vi "Init Deploy.vi"(8 "error in":errorcluster, 10 "Deployment Configuration":T6, 11 "simulator":T2) -> (2 "Communication Refs":T1[](array[typedef]), 3 "Remote Session List":refnum<k21>[](array[refnum]))   [LabVIEW 2014]
uses:
  Deployment  Configuration.ctl
  simulation/Simulator.ctl
  CyberSim interface/Simulation Configuration.ctl
  autograder/feedbackMode.ctl
  RobotData.ctl
  <instrlib>/DC Motor Controller/HAIOL/DC Motor Controller.lvclass
  iRobot Remote Ref.ctl
  iRobot/Sensor/Sensor Group 6.ctl
  iRobot/Sensor/Bumps + Wheel Drops.ctl
  iRobot/Sensor/Buttons.ctl
  iRobot/Sensor/Charging State.ctl
  iRobot/Sensor/Charging Sources Available.ctl
  iRobot/Sensor/OI Mode.ctl
  iRobot/Sensor/Cargo Bay Digital Inputs.ctl
  iRobot/Sensor/Low-Side Driver + Wheel Overcurrent.ctl
  <resource>/objmgr/nisysapi.rc
panel:
  # "Electrical: charging, battery, OI mode"
  # "Sensors: bump, cliff, button, wheel drop, wall, virtual wall"
  # "Motion: distance, angle, requested velocity"
  # "Cargo Bay: I/O, overcurrent, infrared"
  # "Song"
  # "Electrical: charging, battery, OI mode"
  # "Sensors: bump, cliff, button, wheel drop, wall, virtual wall"
  # "Motion: distance, angle, requested velocity"
  # "Cargo Bay: I/O, overcurrent, infrared"
  # "Song"
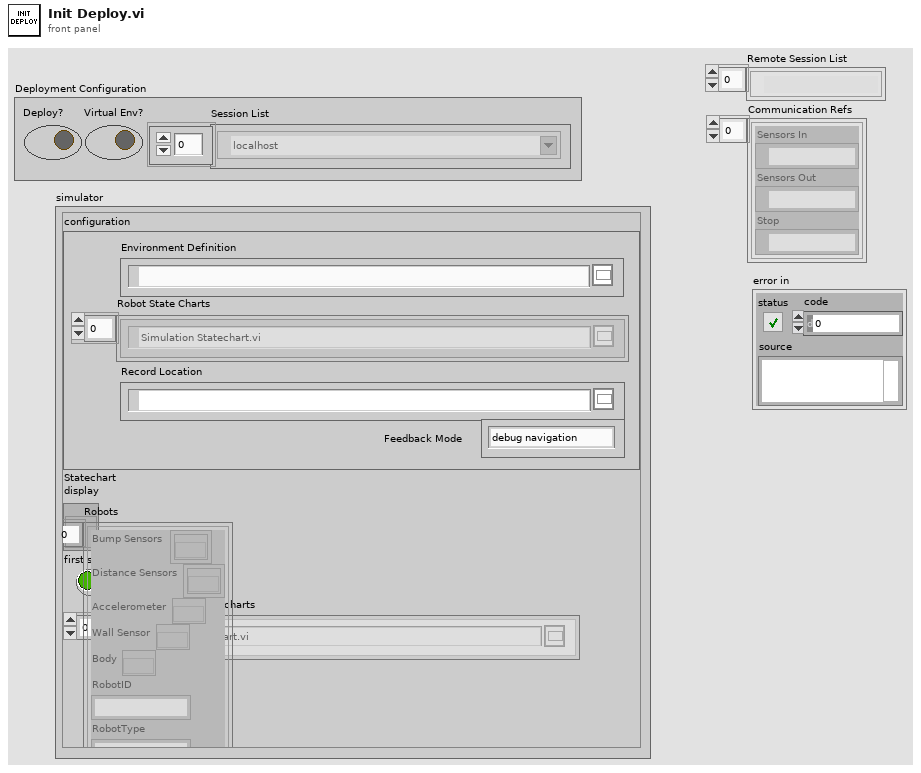
[diagram p1: front panel]
types:
  T1 = typedef "iRobot Remote Ref.ctl" = cluster{"Sensors In":refnum<k21>, "Sensors Out":refnum<k21>, "Stop":refnum<k21>}
  T2 = typedef "Simulator.ctl" = cluster{"configuration":T3, "Statechart\ndisplay":refnum<vi>, "first step?":bool, "Robots Simulation Statecharts":path[], "Robots":T5[]}
  T3 = typedef "Simulation Configuration.ctl" = cluster{"maxTime":sgl, "enableVisualization":bool, "Environment Definition":path, "Record Location":path, "autograde?":bool, "interactive?":bool, "Feedback Mode":T4, "Robot State Charts":path[], "statechart":path}
  T4 = typedef "feedbackMode.ctl" = enum32{"debug navigation", "debug hill climb", "autograde navigation", "autograde hill climb"}
  T5 = typedef "RobotData.ctl" = cluster{"Bump Sensors":refnum<k20>[], "Distance Sensors":refnum<k20>[], "Accelerometer":refnum<k20>, "Wall Sensor":refnum<k20>, "Body":refnum<k20>, "RobotID":string, "RobotType":string, "Left Motor":refnum<class "DC Motor Controller.lvclass">, "Right Motor":refnum<class "DC Motor Controller.lvclass">}
  T6 = typedef "Deployment  Configuration.ctl" = cluster{"Deploy?":bool, "Virtual Env?":bool, "Session List":refnum<k21>[]}
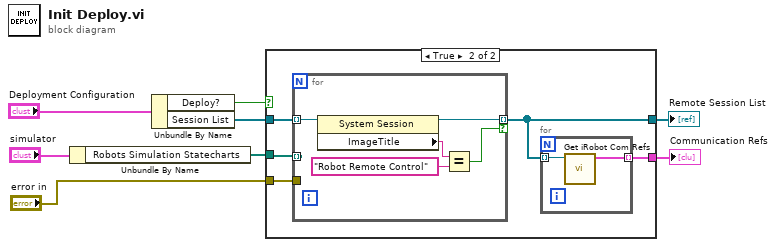
[diagram p0: block diagram]
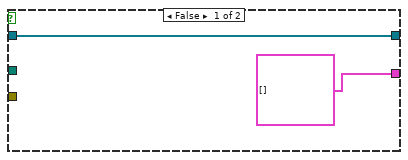
[diagram p2: hidden frame]
diagram:
  n1 = Unbundle By Name("simulator") -> ("Robots Simulation Statecharts"=w4:path[])
  n2 = Unbundle By Name("Deployment Configuration") -> ("Deploy?"=w6:bool, "Session List"=w5:refnum<k21>[])
  n3 = case shown="True" w6 {
    tunnel: w5 -> [w9 w13]
    tunnel: w4 -> [_ w15]
    tunnel: "error in" -> [_ w14]
    tunnel: [w9 w12] -> w2
    tunnel: [T1[] [] w11] -> w1
    frame False {
    }
    frame True {
      n4 = for {
        tunnel: w15 -> [_] mode=indexing
        tunnel: w14 -> [_]
        tunnel: w13 -> [w22] mode=indexing
        tunnel: [w19] -> w12 mode=indexing if=w18
        n5 = property class="System Session"(reference=w22) -> (reference out=w19:refnum<k21>, "ImageTitle"=w20:string)  [unwired: 1 in, 1 out]
        n6 = Equal?(x=w20, y="Robot Remote Control" ("Image Metadata:Title")) -> (x = y?=w18:bool)
      }
      n7 = for {
        tunnel: w12 -> [w17] mode=indexing
        tunnel: [w16] -> w11 mode=indexing
        n8 = call "Get iRobot Com Refs.vi"("Refnum in"=w17) -> ("output cluster"=w16:T1)  [unwired: 10 in]
      }
    }
  }
  "Remote Session List" <- w2
  "Communication Refs" <- w1
